vi "NumericCtlValueCoercion-Test.vi"() -> ()   [LabVIEW 2016]
uses:
  main/apis/Setup/GetVI/GetVIByPath.vi
  main/apis/Stimulus/VI/OpenVIFrontPanel.vi
  main/apis/Stimulus/VI/RunVI.vi
  main/apis/Stimulus/KeyBoardSimulation/Core/KeyBoardSimulation.vi
  main/apis/Assert/AssertControlValue/Equal.vi
  main/apis/Stimulus/KeyBoardSimulation/ValueSignalLatchBooleanString.vi
  main/Drona.lvlib
  main/apis/Setup/GetVI/GetVI.lvlib
  <vilib>/addons/_JKI Toolkits/Caraya/classes/Test/Test.lvclass
  main/apis/Assert/AssertControlValue/AssertControlValue.lvlib
  main/apis/Stimulus/KeyBoardSimulation/KeyboardSimulation.lvlib
  main/apis/Stimulus/VI/VI.lvlib
panel:
  out "error out":errorcluster
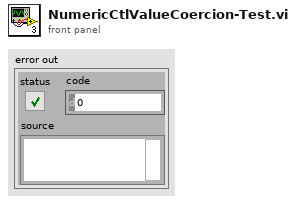
[diagram p1: front panel]
types:
  T1 = cluster{" Key":u8, "Action":enum16{"Press", "Up", "Down"}, "Delay (ms)":u32}[]
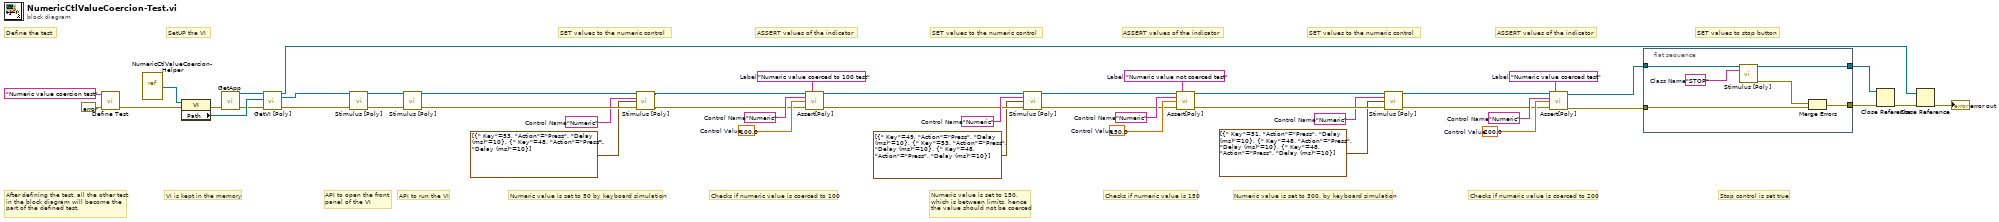
[diagram p0: block diagram]
diagram:
  (unwired) T1 [{" Key"=53, "Action"=enum."Press", "Delay (ms)"=10}, {" Key"=48, "Action"=enum."Press", "Delay (ms)"=10}] ("Key Array")
  w19 = "Numeric"  # Control Name
  w20 = "Numeric value coerced test"  # Label
  w21 = 200.0  # Control Value
  w6 = "Numeric"  # Control Name
  w36 = "Numeric"  # Control Name
  w34 = "Numeric value not coerced test"  # Label
  w33 = 150.0  # Control Value
  w35 = "Numeric"  # Control Name
  w37 = "Numeric"  # Control Name
  w38 = "Numeric value coerced to 100 test"  # Label
  w39 = 100.0  # Control Value
  w8 = "Numeric"  # Control Name
  # "Checks if numeric value is coerced to 200"
  # "ASSERT values of the indicator"
  # "Numeric value is set to 300, by keyboard simulation"
  # "SET values to the numeric control"
  # "API to open the front\npanel of the VI"
  # "Stop control is set true"
  # "SET values to stop button"
  # "Checks if numeric value is 150"
  # "ASSERT values of the indicator"
  # "Numeric value is set to 150, \nwhich is between limits, hence\nthe value should not be coerced"
  # "SET values to the numeric control"
  # "Checks if numeric value is coerced to 100"
  # "ASSERT values of the indicator"
  # "Numeric value is set to 50 by keyboard simulation"
  # "API to run the VI"
  # "SET values to the numeric control"
  # "VI is kept in the memory"
  # "SetUP the VI"
  # "After defining the test, all the other test\nin the block diagram will become the \npart of the defined test."
  # "Define the test"
  n1 = call <vilib>:"Define Test.vi"("error in (no error)"=errorcluster {"status"=FALSE, "code"=0, "source"=""}, "Label (VI Title)"="Numeric value coercion test") -> ("error out"=w41:errorcluster)  [unwired: 9 in]
  n2 = vi-ref "NumericCtlValueCoercion-Helper.vi"() -> (w1:refnum<vi>)
  n3 = property on="Property Node" class="VI"(reference=w1, error in=w41) -> (error out=w45:errorcluster, "Path"=w44:path)  [unwired: 1 out]
  n4 = call "GetApp.vi"("error in (no error)"=w45) -> ("Application Ref"=w46:refnum<vi>, "error out"=w43:errorcluster)  [unwired: 13 in]
  n5 = call-poly "GetVI [Poly].vi"("Application Ref in"=w46, "VI Path"=w44, "error in (no error)"=w43) -> ("Application Ref out"=w2:refnum<vi>, "VI Reference"=w25:refnum<vi>, "error out"=w27:errorcluster)  [unwired: 10 in]
  n6 = call-poly "Stimulus [Poly].vi"("VI Reference In"=w25, "error in"=w27) -> ("VI Reference Out"=w24:refnum<vi>, "error out"=w26:errorcluster)  [unwired: 12 in]
  n7 = call-poly "Stimulus [Poly].vi"("VI Reference In"=w24, "error in"=w26) -> ("VI Reference Out"=w15:refnum<vi>, "error out"=w16:errorcluster)  [unwired: 12 in]
  n8 = call-poly "Stimulus [Poly].vi"("VI Reference In"=w15, "Control Path"=w8, "Key Array"=T1 [{" Key"=53, "Action"=enum."Press", "Delay (ms)"=10}, {" Key"=48, "Action"=enum."Press", "Delay (ms)"=10}], "error In"=w16) -> ("VI Reference Out"=w14:refnum<vi>, "error IO"=w13:errorcluster)  [unwired: 10 in]
  n9 = call-poly "Assert[Poly].vi"("VI Reference In"=w14, "Label"=w38, "Control Path"=w37, "Control Value"=w39, "Error In"=w13) -> ("VI Reference Out"=w29:refnum<vi>, "Error Out"=w30:errorcluster)  [unwired: 9 in]
  n10 = call-poly "Stimulus [Poly].vi"("VI Reference In"=w29, "Control Path"=w35, "Key Array"=T1 [{" Key"=49, "Action"=enum."Press", "Delay (ms)"=10}, {" Key"=53, "Action"=enum."Press", "Delay (ms)"=10}, {" Key"=48, "Action"=enum."Press", "Delay (ms)"=10}], "error In"=w30) -> ("VI Reference Out"=w32:refnum<vi>, "error IO"=w31:errorcluster)  [unwired: 10 in]
  n11 = call-poly "Assert[Poly].vi"("VI Reference In"=w32, "Label"=w34, "Control Path"=w36, "Control Value"=w33, "Error In"=w31) -> ("VI Reference Out"=w11:refnum<vi>, "Error Out"=w12:errorcluster)  [unwired: 9 in]
  n12 = call-poly "Stimulus [Poly].vi"("VI Reference In"=w11, "Control Path"=w6, "Key Array"=T1 [{" Key"=51, "Action"=enum."Press", "Delay (ms)"=10}, {" Key"=48, "Action"=enum."Press", "Delay (ms)"=10}, {" Key"=48, "Action"=enum."Press", "Delay (ms)"=10}], "error In"=w12) -> ("VI Reference Out"=w10:refnum<vi>, "error IO"=w9:errorcluster)  [unwired: 10 in]
  n13 = call-poly "Assert[Poly].vi"("VI Reference In"=w10, "Label"=w20, "Control Path"=w19, "Control Value"=w21, "Error In"=w9) -> ("VI Reference Out"=w17:refnum<vi>, "Error Out"=w18:errorcluster)  [unwired: 9 in]
  n14 = flat-sequence {
    tunnel: [w50] -> w23
    tunnel: [w51] -> w22
    tunnel: w17 -> [w49]
    tunnel: w18 -> [w47]
    frame #0 {
      w52 = "STOP"  # Class Name
      n15 = call-poly "Stimulus [Poly].vi"("VI Reference In"=w49, "Control Path"=w52) -> ("VI Reference Out"=w51:refnum<vi>, "error out"=w48:errorcluster)  [unwired: 12 in]
      n16 = Merge Errors(w48, w47) -> (w50:errorcluster)
    }
  }
  n17 = Close Reference(reference=w22, error in (no error)=w23) -> (error out=w28:errorcluster)
  n18 = Close Reference(reference=w2, error in (no error)=w28) -> (error out=→"error out":errorcluster)
